vi "FCI BIN Coord.vi"(0 "Image In":T1(plugin-control), 11 "error in (no error)":errorcluster) -> (4 "Image Out":T1, 6 "Coord details":T2, 15 "error IO":errorcluster)   [LabVIEW 2019, in "Algorithm.lvclass"]
uses:
  FrameworkOverrides/Algorithm.lvclass
  <vilib>/vision/NI_Vision_Development_Module.lvlib
  <vilib>/vision/Measure.llb/Straight Edge Process.ctl
  <vilib>/vision/Measure.llb/Straight Edge Options.ctl
  <vilib>/vision/Measure.llb/Edge Polarity.ctl
  <vilib>/vision/Measure.llb/Edge Options.ctl
  <vilib>/vision/Image Controls.llb/IMAQ Image.ctl
panel:
  in  "Y coord lower limit":dbl=350.0 format="%#_13g"
  in  "Y coord upper limit":dbl=730.0 format="%#_13g"
  out "Y Coord":dbl[](array[numeric])
  out "Number of Particles":i32
  out "subarray 2":dbl[](array[numeric])
  out "index of element":i32
  out "Array":bool[](array[boolean])
  out "X Coord":dbl[](array[numeric])
  out "Image 2":T1(plugin-control)
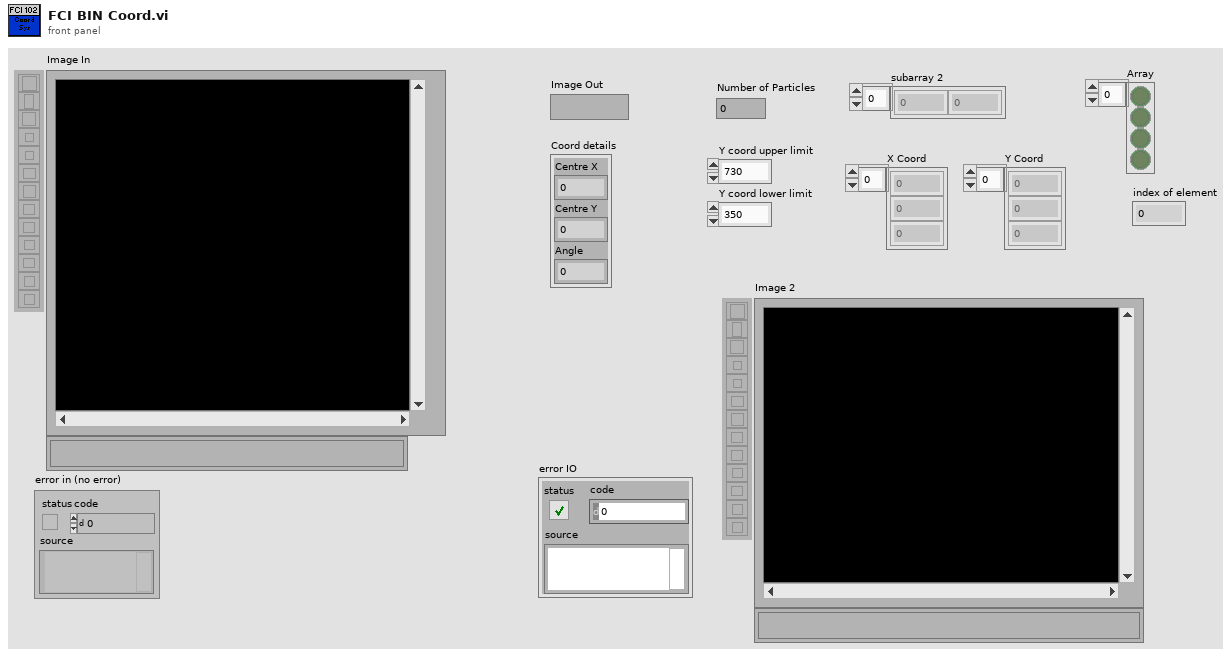
[diagram p1: front panel]
types:
  T1 = typedef "IMAQ Image.ctl" = refnum<image>
  T2 = cluster{"Centre X":dbl, "Centre Y":dbl, "Angle":dbl}
  T3 = cluster{"Left":dbl, "Top":dbl, "Right":dbl, "Bottom":dbl, "Angle":dbl}
  T4 = typedef "Edge Options.ctl" = cluster{"Edge Polarity":T5, "Kernel Size":u32, "Width":u32, "Minimum Edge Strength":sgl, "Interpolation Type":enum32{"Zero Order", "Bilinear", "Quadratic", "Cubic", "Bilinear Fixed"}, "Data Processing Method":enum32{"Average", "Median"}}
  T5 = typedef "Edge Polarity.ctl" = u32
  T6 = cluster{"Search Direction":u32, "Edge Options":T4, "Show Search Area":bool, "Show Search Lines":bool, "Show Edges Found":bool, "Show Result":bool, "Search Area Color":u32, "Search Lines Color":u32, "Edge Locations Color":u32, "Result Color":u32, "Overlay Group Name":string}
  T7 = typedef "Straight Edge Options.ctl" = cluster{"Number of Lines":i32, "Type":T8, "Min. Score":dbl, "Max. Score":dbl, "Orientation":dbl, "Angle Range":dbl, "Angle Tolerance":dbl, "Step Size":u32, "Min. SNR (db)":dbl, "Min. Points (%)":dbl, "Hough Iterations":i32}
  T8 = typedef "Straight Edge Process.ctl" = enum32{"First Edge Rake", "Best Edge Rake", "Hough Edge Rake", "First Edge Projection", "Best Edge Projection"}
  T9 = typedef "Particle Parameters" = i32
  T10 = cluster{"Measurement Parameter":T9, "Range Lower Value":dbl, "Range Upper Value":dbl, "Range":bool, "Measurement Type":bool}[]
  T11 = typedef "Image Type" = u32
  T12 = typedef "ROI Descriptor" = cluster{"Global Rectangle":i32[], "Contours":cluster{"ID":enum32{"External", "Internal"}, "Type":u32, "Coordinates":i32[]}[]}
  T13 = cluster{"Point1 (Pixels)":cluster{"X":sgl, "Y":sgl}, "Point2 (Pixels)":cluster{"X":sgl, "Y":sgl}, "Point1 (Real-World)":cluster{"X":sgl, "Y":sgl}, "Point2 (Real-World)":cluster{"X":sgl, "Y":sgl}, "Angle (Pixel)":dbl, "Angle (Real-World)":dbl, "Score":dbl, "Straightness":dbl, "Average SNR (db)":dbl, "Calibration Valid":bool}[]
  T14 = cluster{"Point1 (Pixels)":cluster{"X":sgl, "Y":sgl}, "Point2 (Pixels)":cluster{"X":sgl, "Y":sgl}, "Point1 (Real-World)":cluster{"X":sgl, "Y":sgl}, "Point2 (Real-World)":cluster{"X":sgl, "Y":sgl}, "Angle (Pixel)":dbl, "Angle (Real-World)":dbl, "Score":dbl, "Straightness":dbl, "Average SNR (db)":dbl, "Calibration Valid":bool}
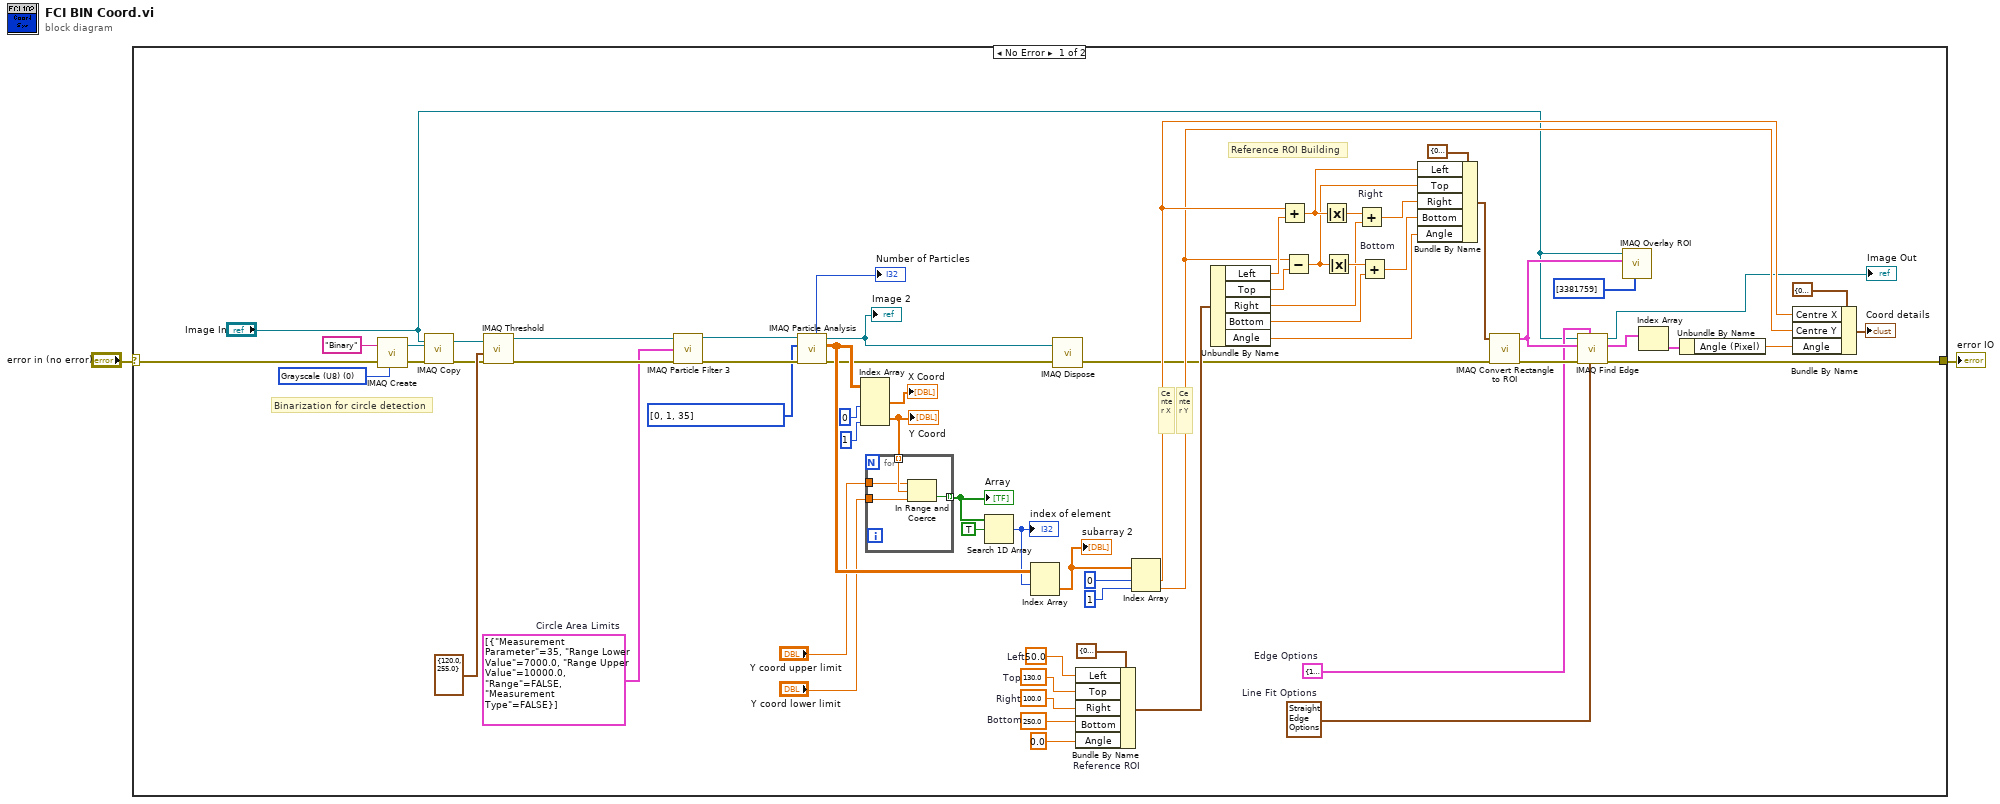
[diagram p0: block diagram]
diagram:
  n1 = case shown="No Error" "error in (no error)" {
    selector: "error in (no error)" -> [w7 w73]
    tunnel: [w8 w73] -> w1
    frame No Error {
      w17 = T6 {"Search Direction"=1, "Edge Options"={"Edge Polarity"=0, "Kernel Size"=3, "Width"=3, "Minimum Edge Strength"=50.0, "Interpolation Type"=enum."Zero Order", "Data Processing Method"=enum."Average"}, "Show Search Area"=FALSE, "Show Search Lines"=FALSE, "Show Edges Found"=FALSE, "Show Result"=TRUE, "Search Area Color"=65280, "Search Lines Color"=255, "Edge Locations Color"=16776960, "Result Color"=16711680, "Overlay Group Name"=""}  # Edge Options
      w46 = T7 {"Number of Lines"=1, "Type"=enum."First Edge Rake", "Min. Score"=10.0, "Max. Score"=1000.0, "Orientation"=0.0, "Angle Range"=45.0, "Angle Tolerance"=1.0, "Step Size"=3, "Min. SNR (db)"=0.0, "Min. Points (%)"=25.0, "Hough Iterations"=5}  # Line Fit Options
      w24 = 250.0  # Bottom
      w25 = 100.0  # Right
      w26 = 130.0  # Top
      w27 = 50.0  # Left
      w60 = T9[] [0, 1, 35] items=["Center of Mass X", "Center of Mass Y", "First Pixel X", "First Pixel Y", "Bounding Rect Left", "Bounding Rect Top", "Bounding Rect Right", "Bounding Rect Bottom", "Max Feret Diameter Start X", "Max Feret Diameter Start Y", "Max Feret Diameter End X", "Max Feret Diameter End Y", "Max Horiz. Segment Length Left", "Max Horiz. Segment Length Right", "Max Horiz. Segment Length Row", "-", "Bounding Rect Width", "Bounding Rect Height", "Bounding Rect Diagonal", "Perimeter", "Convex Hull Perimeter", "Holes' Perimeter", "Max Feret Diameter", "Equivalent Ellipse Major Axis", "Equivalent Ellipse Minor Axis", "Equivalent Ellipse Minor Axis (Feret)", "Equivalent Rect Long Side", "Equivalent Rect Short Side", "Equivalent Rect Diagonal", "Equivalent Rect Short Side (Feret)", "Average Horiz. Segment Length", "Average Vert. Segment Length", "Hydraulic Radius", "Waddel Disk Diameter", "-", "Area", "Holes' Area", "Particle & Holes' Area", "Convex Hull Area", "Image Area", "-", "Number of Holes", "Number of Horiz. Segments", "Number of Vert. Segments", "-", "Orientation", "Max Feret Diameter Orientation", "-", "% Area/Image Area", "% Area/(Particle & Holes' Area)", "Ratio of Equivalent Ellipse Axes", "Ratio of Equivalent Rect Sides", "-", "Elongation Factor", "Compactness Factor", "Heywood Circularity Factor", "Type Factor", "-", "Sum X", "Sum Y", "Sum XX", "Sum XY", "Sum YY", "Sum XXX", "Sum XXY", "Sum XYY", "Sum YYY", "-", "Moment of Inertia XX", "Moment of Inertia XY", "Moment of Inertia YY", "Moment of Inertia XXX", "Moment of Inertia XXY", "Moment of Inertia XYY", "Moment of Inertia YYY", "Norm. Moment of Inertia XX", "Norm. Moment of Inertia XY", "Norm. Moment of Inertia YY", "Norm. Moment of Inertia XXX", "Norm. Moment of Inertia XXY", "Norm. Moment of Inertia XYY", "Norm. Moment of Inertia YYY", "Hu Moment 1", "Hu Moment 2", "Hu Moment 3", "Hu Moment 4", "Hu Moment 5", "Hu Moment 6", "Hu Moment 7"] ("Pixel Measurements")
      w19 = T10 [{"Measurement Parameter"=35, "Range Lower Value"=7000.0, "Range Upper Value"=10000.0, "Range"=FALSE, "Measurement Type"=FALSE}]  # Circle Area Limits
      w67 = T11 0 items=["Grayscale (U8)", "Grayscale (I16)", "Grayscale (SGL)", "Complex (CSG)", "RGB (U32)", "HSL (U32)", "RGB (U64)", "Grayscale (U16)"] ("Image Type")
      # "Binarization for circle detection"
      # "Reference ROI Building"
      # "Center Y"
      # "Center X"
      n2 = call "IMAQ Create"("Image Name"="Binary", "Image Type"=w67, "error in (no error)"=w7) -> ("New Image"=w66:T1, "error out"=w65:errorcluster)  [unwired: 2 in]
      n3 = call "IMAQ Copy"("error in (no error)"=w65, "Image Dst"=w66, "Image Src"="Image In") -> ("error out"=w18:errorcluster, "Image Dst Out"=w42:T1)  [unwired: 3 in]
      n4 = call "IMAQ Threshold"("error in (no error)"=w18, "Range"=cluster{"Lower value":sgl, "Upper value":sgl} {"Lower value"=120.0, "Upper value"=255.0}, "Image Src"=w42) -> ("error out"=w64:errorcluster, "Image Dst Out"=w63:T1)  [unwired: 7 in]
      n5 = call "IMAQ Particle Filter 3"("Image Src"=w63, "Selection Values"=w19, "error in (no error)"=w64) -> ("Image Dst Out"=w62:T1, "error out"=w61:errorcluster)  [unwired: 10 in, 1 out]
      n6 = call "IMAQ Particle Analysis"("error in (no error)"=w61, "Pixel Measurements"=w60, "Image"=w62) -> ("error out"=w5:errorcluster, "Particle Measurements (Pixels)"=w38:dbl[][], "Image Out (duplicate)"=w3:T1, "Number of Particles"=→"Number of Particles":i32)  [unwired: 3 in, 2 out]
      "Image 2" <- w3
      n7 = Index Array(array=w38, index (col) #1=0 ("disabled index (col)"), index (col) #2=1 ("index (col)")) -> (element #1=→"X Coord":dbl[], element #2=w30:dbl[])  [unwired: 2 in]
      "Y Coord" <- w30
      n8 = for {
        tunnel: w30 -> [w72] mode=indexing
        tunnel: [w71] -> w40 mode=indexing
        tunnel: "Y coord upper limit" -> [w70]
        tunnel: "Y coord lower limit" -> [w69]
        n9 = In Range and Coerce(upper limit=w70, x=w72, lower limit=w69) -> (In Range?=w71:bool)  [unwired: 1 out]
      }
      "Array" <- w40
      n10 = Search 1D Array(1D array=w40, element=TRUE) -> (index of element=w37:i32)  [unwired: 1 in]
      "index of element" <- w37
      n11 = Index Array(array=w38, index (row)=w37) -> (element=w36:dbl[])  [unwired: 1 in]
      "subarray 2" <- w36
      n12 = call "IMAQ Dispose"("Image"=w3, "error in (no error)"=w5) -> ("error out"=w4:errorcluster)  [unwired: 4 in]
      n13 = Bundle By Name "Reference ROI"(cluster=T3 {"Left"=0.0, "Top"=0.0, "Right"=0.0, "Bottom"=0.0, "Angle"=0.0} ("input cluster"), "Left"=w27, "Top"=w26, "Right"=w25, "Bottom"=w24, "Angle"=0.0) -> (w15:T3)
      n14 = Index Array(array=w36, index #1=0 ("index"), index #2=1 ("index")) -> (element #1=w13:dbl, element #2=w12:dbl)
      n15 = Unbundle By Name(w15) -> ("Left"=w52:dbl, "Top"=w51:dbl, "Right"=w50:dbl, "Bottom"=w49:dbl, "Angle"=w48:dbl)
      n16 = Add(x=w13, y=w52) -> (x+y=w56:dbl)
      n17 = Subtract(x=w12, y=w51) -> (x-y=w55:dbl)
      n18 = Absolute Value(x=w56) -> (abs(x)=w59:dbl)
      n19 = Absolute Value(x=w55) -> (abs(x)=w58:dbl)
      n20 = Add "Right"(x=w59, y=w50) -> (x+y=w54:dbl)
      n21 = Add "Bottom"(x=w58, y=w49) -> (x+y=w53:dbl)
      n22 = Bundle By Name(cluster=T3 {"Left"=0.0, "Top"=0.0, "Right"=0.0, "Bottom"=0.0, "Angle"=0.0} ("input cluster"), "Left"=w56, "Top"=w55, "Right"=w54, "Bottom"=w53, "Angle"=w48) -> (w43:T3)
      n23 = call "IMAQ Convert Rectangle to ROI"("error in (no error)"=w4, "Rectangle"=w43) -> ("error out"=w47:errorcluster, "ROI Descriptor"=w21:T12)  [unwired: 7 in]
      n24 = call "IMAQ Find Edge"("Line Fit Options"=w46, "Options"=w17, "error in (no error)"=w47, "ROI Descriptor"=w21, "Image"="Image In") -> ("error out"=w8:errorcluster, "Straight Edges"=w45:T13, "Image Out"=→"Image Out":T1)  [unwired: 3 in, 1 out]
      n25 = call "IMAQ Overlay ROI"("Colors (Green)"=u32[] [3381759], "ROI Descriptor"=w21, "Image"="Image In") -> ()  [unwired: 7 in, 2 out]
      n26 = Index Array(array=w45) -> (element=w44:T14)  [unwired: 1 in]
      n27 = Unbundle By Name(w44) -> ("Angle (Pixel)"=w14:dbl)
      n28 = Bundle By Name(cluster=T2 {"Centre X"=0.0, "Centre Y"=0.0, "Angle"=0.0} ("output cluster"), "Centre X"=w13, "Centre Y"=w12, "Angle"=w14) -> (→"Coord details":T2)
    }
    frame Error {
    }
  }
  "error IO" <- w1
